vi "graph_data.vi"(0 "Notifier in":refnum<notifier>, 1 "X":T1 items=["DSRED"=30, "TIME"=0, "FSC"=1, "SSC"=6, "FITC"=9], 2 "Y":T1 items=["DSRED"=30, "TIME"=0, "FSC"=1, "SSC"=6, "FITC"=9], 3 "Reactor to display":i32) -> (7 "Notifier in 2":refnum<notifier>, 8 "Cluster":T3, 9 "Histogram":dynamicdata(waveform), 10 "SUMMARY STATS GRAPH":dbl[](array[numeric]))   [LabVIEW 2013]
uses:
  main_machine/type_defs/reactor.ctl
  main_machine/type_defs/reactors.ctl
  main_machine/type_defs/fsc_parameter.ctl
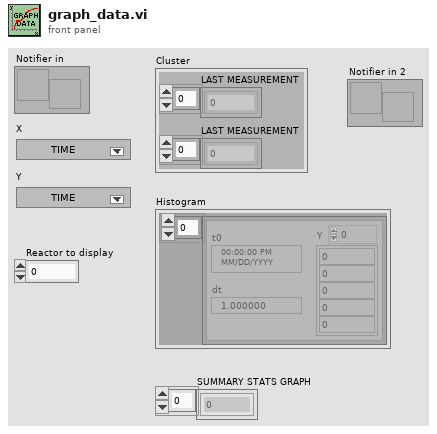
[diagram p1: front panel]
types:
  T1 = typedef "fsc_parameter.ctl" = u16
  T2 = typedef "reactor.ctl" = dbl
  T3 = cluster{"LAST MEASUREMENT":T2[], "LAST MEASUREMENT":T2[]}
  T4 = typedef "reactors.ctl" = cluster{i32, "TIME STAMPS":dbl[], "LAST MEASUREMENT":T2[][], "SUMMARY STAT":dbl[]}[]
  T5 = cluster{i32, "TIME STAMPS":dbl[], "LAST MEASUREMENT":T2[][], "SUMMARY STAT":dbl[]}
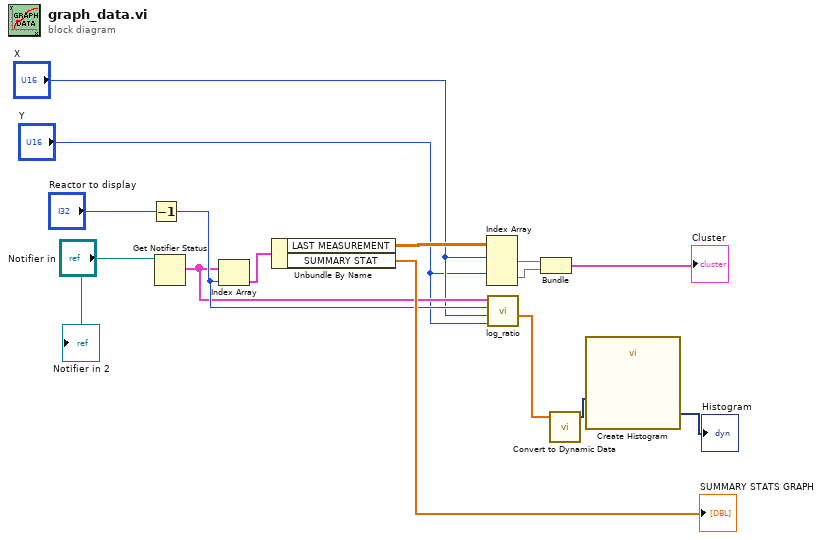
[diagram p0: block diagram]
diagram:
  n1 = Decrement(x="Reactor to display") -> (x-1=w11:i32)
  n2 = Get Notifier Status(notifier="Notifier in") -> (current notification=w10:T4)  [unwired: 1 in, 4 out]
  n3 = Index Array(array=w10, index=w11) -> (element=w3:T5)
  n4 = Unbundle By Name(w3) -> ("LAST MEASUREMENT"=w6:T2[][], "SUMMARY STAT"=→"SUMMARY STATS GRAPH":dbl[])
  n5 = Index Array(array=w6, index (row) #1="X", index (row) #2="Y") -> (element #1=w7:T2[], element #2=w8:T2[])  [unwired: 2 in]
  n6 = call "log_ratio.vi"("Y"="Y", "X"="X", "Reactor (INDEX)"=w11, "REACTORS"=w10) -> ("logratio"=w13:T2[])  [unwired: 5 in, 2 out]
  n7 = Bundle("LAST MEASUREMENT"=w7, "LAST MEASUREMENT"=w8) -> (→"Cluster":T3)  [unwired: 1 in]
  n8 = call "Convert to Dynamic Data"("Array"=w13) -> ("Dynamic Data Type"=w14:dynamicdata)  [unwired: 3 in]
  n9 = call "Create Histogram"("Signal"=w14) -> ("Histogram"=→"Histogram":dynamicdata)  [unwired: 9 in, 1 out]
  "Notifier in 2" <- "Notifier in"
